vi "splitString.vi"(11 "Numeric":u16) -> (1 "hex 3":u8 format="%x", 2 "hex 1":u8 format="%x", 3 "hex 0":u8 format="%x")   [LabVIEW 2013]
panel:
  out "String":string
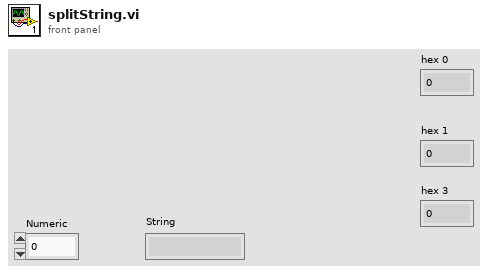
[diagram p1: front panel]
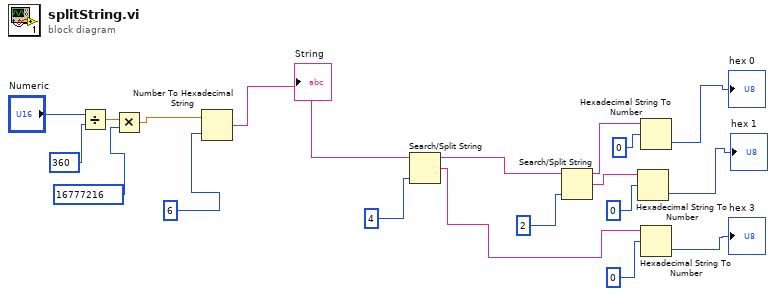
[diagram p0: block diagram]
diagram:
  n1 = Divide(x="Numeric", y=360) -> (x/y=w3:dbl)
  n2 = Multiply(x=w3, y=16777216) -> (x*y=w1:dbl)
  n3 = Number To Hexadecimal String(1:6, 2:w1) -> (0:w18:string)
  "String" <- w18
  n4 = Search/Split String(string=w18, offset (0)=4) -> (substring before match=w16:string, match + rest of string=w11:string)  [unwired: 1 in, 1 out]
  n5 = Search/Split String(string=w16, offset (0)=2) -> (substring before match=w14:string, match + rest of string=w12:string)  [unwired: 1 in, 1 out]
  n6 = Hexadecimal String To Number(string=w12, offset=0) -> (number=→"hex 1":u32)  [unwired: 1 in, 1 out]
  n7 = Hexadecimal String To Number(string=w14, offset=0) -> (number=→"hex 0":u32)  [unwired: 1 in, 1 out]
  n8 = Hexadecimal String To Number(string=w11, offset=0) -> (number=→"hex 3":u32)  [unwired: 1 in, 1 out]
